vi "界面UI.vi"() -> ()   [LabVIEW 2016, in "德润DR803L超标留样.lvlib"]
uses:
  <vilib>/Utility/miscctls.llb/LVPointTypeDef.ctl
  <vilib>/Utility/config.llb/NI_LVConfig.lvlib
  <vilib>/ptbypt/NI_PtbyPt.lvlib
panel:
  in  "超标浓度配置":bool
  out "流程中":bool
  in  "停止流程":bool
  in  "启动流程":bool
  in  "时间等比采样":u16=10
  in  "单次采样量":u16=500
  in  "修改门禁密码":bool
  in  "远程复位":bool
  in  "排空当前瓶":bool
  in  "采样方式":enum16{"单采", "双重"}(ring)
  in  "远程留样":bool
  in  "选择留样瓶":bool
  in  "排空留样瓶":bool
  out "采样器状态":T1
  out "Registers":u16[](array[numeric])
  in  "打开串口":bool
  in  "释放串口":bool
  in  "留样模式":T2(ring)=enum."外控留样"
  in  "采样启动":bool
  in  "停止命令":bool
  in  "切换采样器状态":bool
  in  "时间校准":bool
  out "source":string
  out "通讯":bool
  # "只在停止时切换有效"
  # "只在待机时切换有效"
  # "默认：500ml（5-1000）ml （只在停止时写有效）"
  # "只在待机时启动有效"
  # "默认：10min（2-9999）min （只在停止时写有效）"
  # "只在待机时启动有效"
  # "只在待机时启动有效"
  # "德润DR803L超标留样"
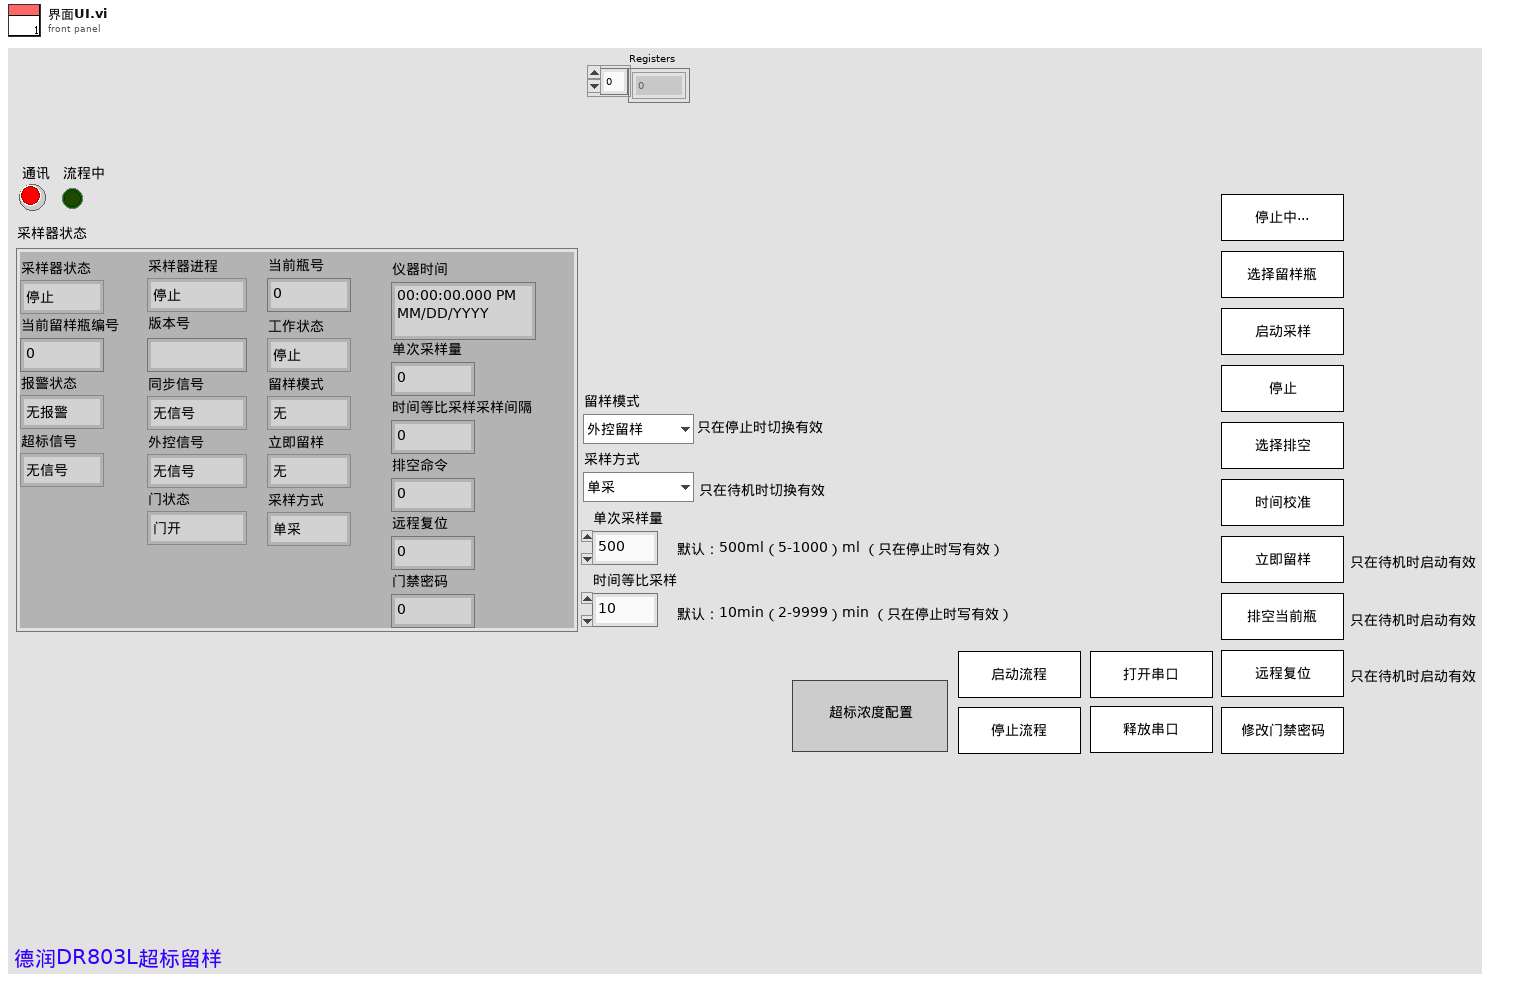
[diagram p1: front panel]
types:
  T1 = cluster{"采样器状态":enum16{"停止", "运行"}, "当前留样瓶编号":u16, "报警状态":enum16{"无报警", "缺水报警"}, "超标信号":enum16{"无信号", "超标信号"}, "采样器进程":enum16{"停止", "待机", "定位校正", "移除瓶盖", "采样瓶排空", "管路润洗", "管存", "进样", "瓶盖密封", "管路排空", "调整采样位置", "采样结束", "采样瓶润洗", "瓶润洗排空"}, "版本号":string, "同步信号":enum16{"无信号", "同步信号"}, "外控信号":enum16{"无信号", "外控信号"}, "门状态":enum16{"门开", "门关"}, "当前瓶号":u16, "工作状态":enum16{"停止", "采样中"}, "留样模式":enum16{"无", "定时留样", "时间等比例", "超标留样", "同步留样", "外控留样"}, "立即留样":enum16{"无", "远程留样"}, "采样方式":enum16{"单采", "双重"}, "仪器时间":timestamp, "单次采样量":u16, "时间等比采样采样间隔":u16, "排空命令":u16, "远程复位":u16, "门禁密码":u16}
  T2 = enum16{"无", "定时留样", "时间等比例", "超标留样", "同步留样", "外控留样"}
  T3 = cluster{"STEP":enum16{"open", "read", "write", "write single", "close"}, "starting address":u16, "value":u16}
  T4 = typedef "LVPointTypeDef.ctl" = cluster{"Horizontal":i16, "Vertical":i16}
  T5 = typedef "NI_LVConfig.lvlib/Config Data RefNum.ctl" = refnum<k1>
  T6 = enum16{"open", "read", "write", "write single", "close"}
  T7 = cluster{"氨氮超标浓度":dbl, "总磷超标浓度":dbl, "总氮超标浓度":dbl, "CODMn超标浓度":dbl, "CODCr超标浓度":dbl}
  T8 = typedef "LVDateTimeRec.ctl" = cluster{"秒数的小数部分":dbl, "秒":i32, "分":i32, "时":i32, "日":i32, "月":i32, "年":i32, "天数（周）":i32, "天数（年）":i32, "DST":i32}
  T9 = enum32{"Bad", "Idle", "Run top level", "Running"}
  T10 = cluster{"确定":bool, "氨氮超标浓度":dbl, "总磷超标浓度":dbl, "总氮超标浓度":dbl, "CODMn超标浓度":dbl, "CODCr超标浓度":dbl}
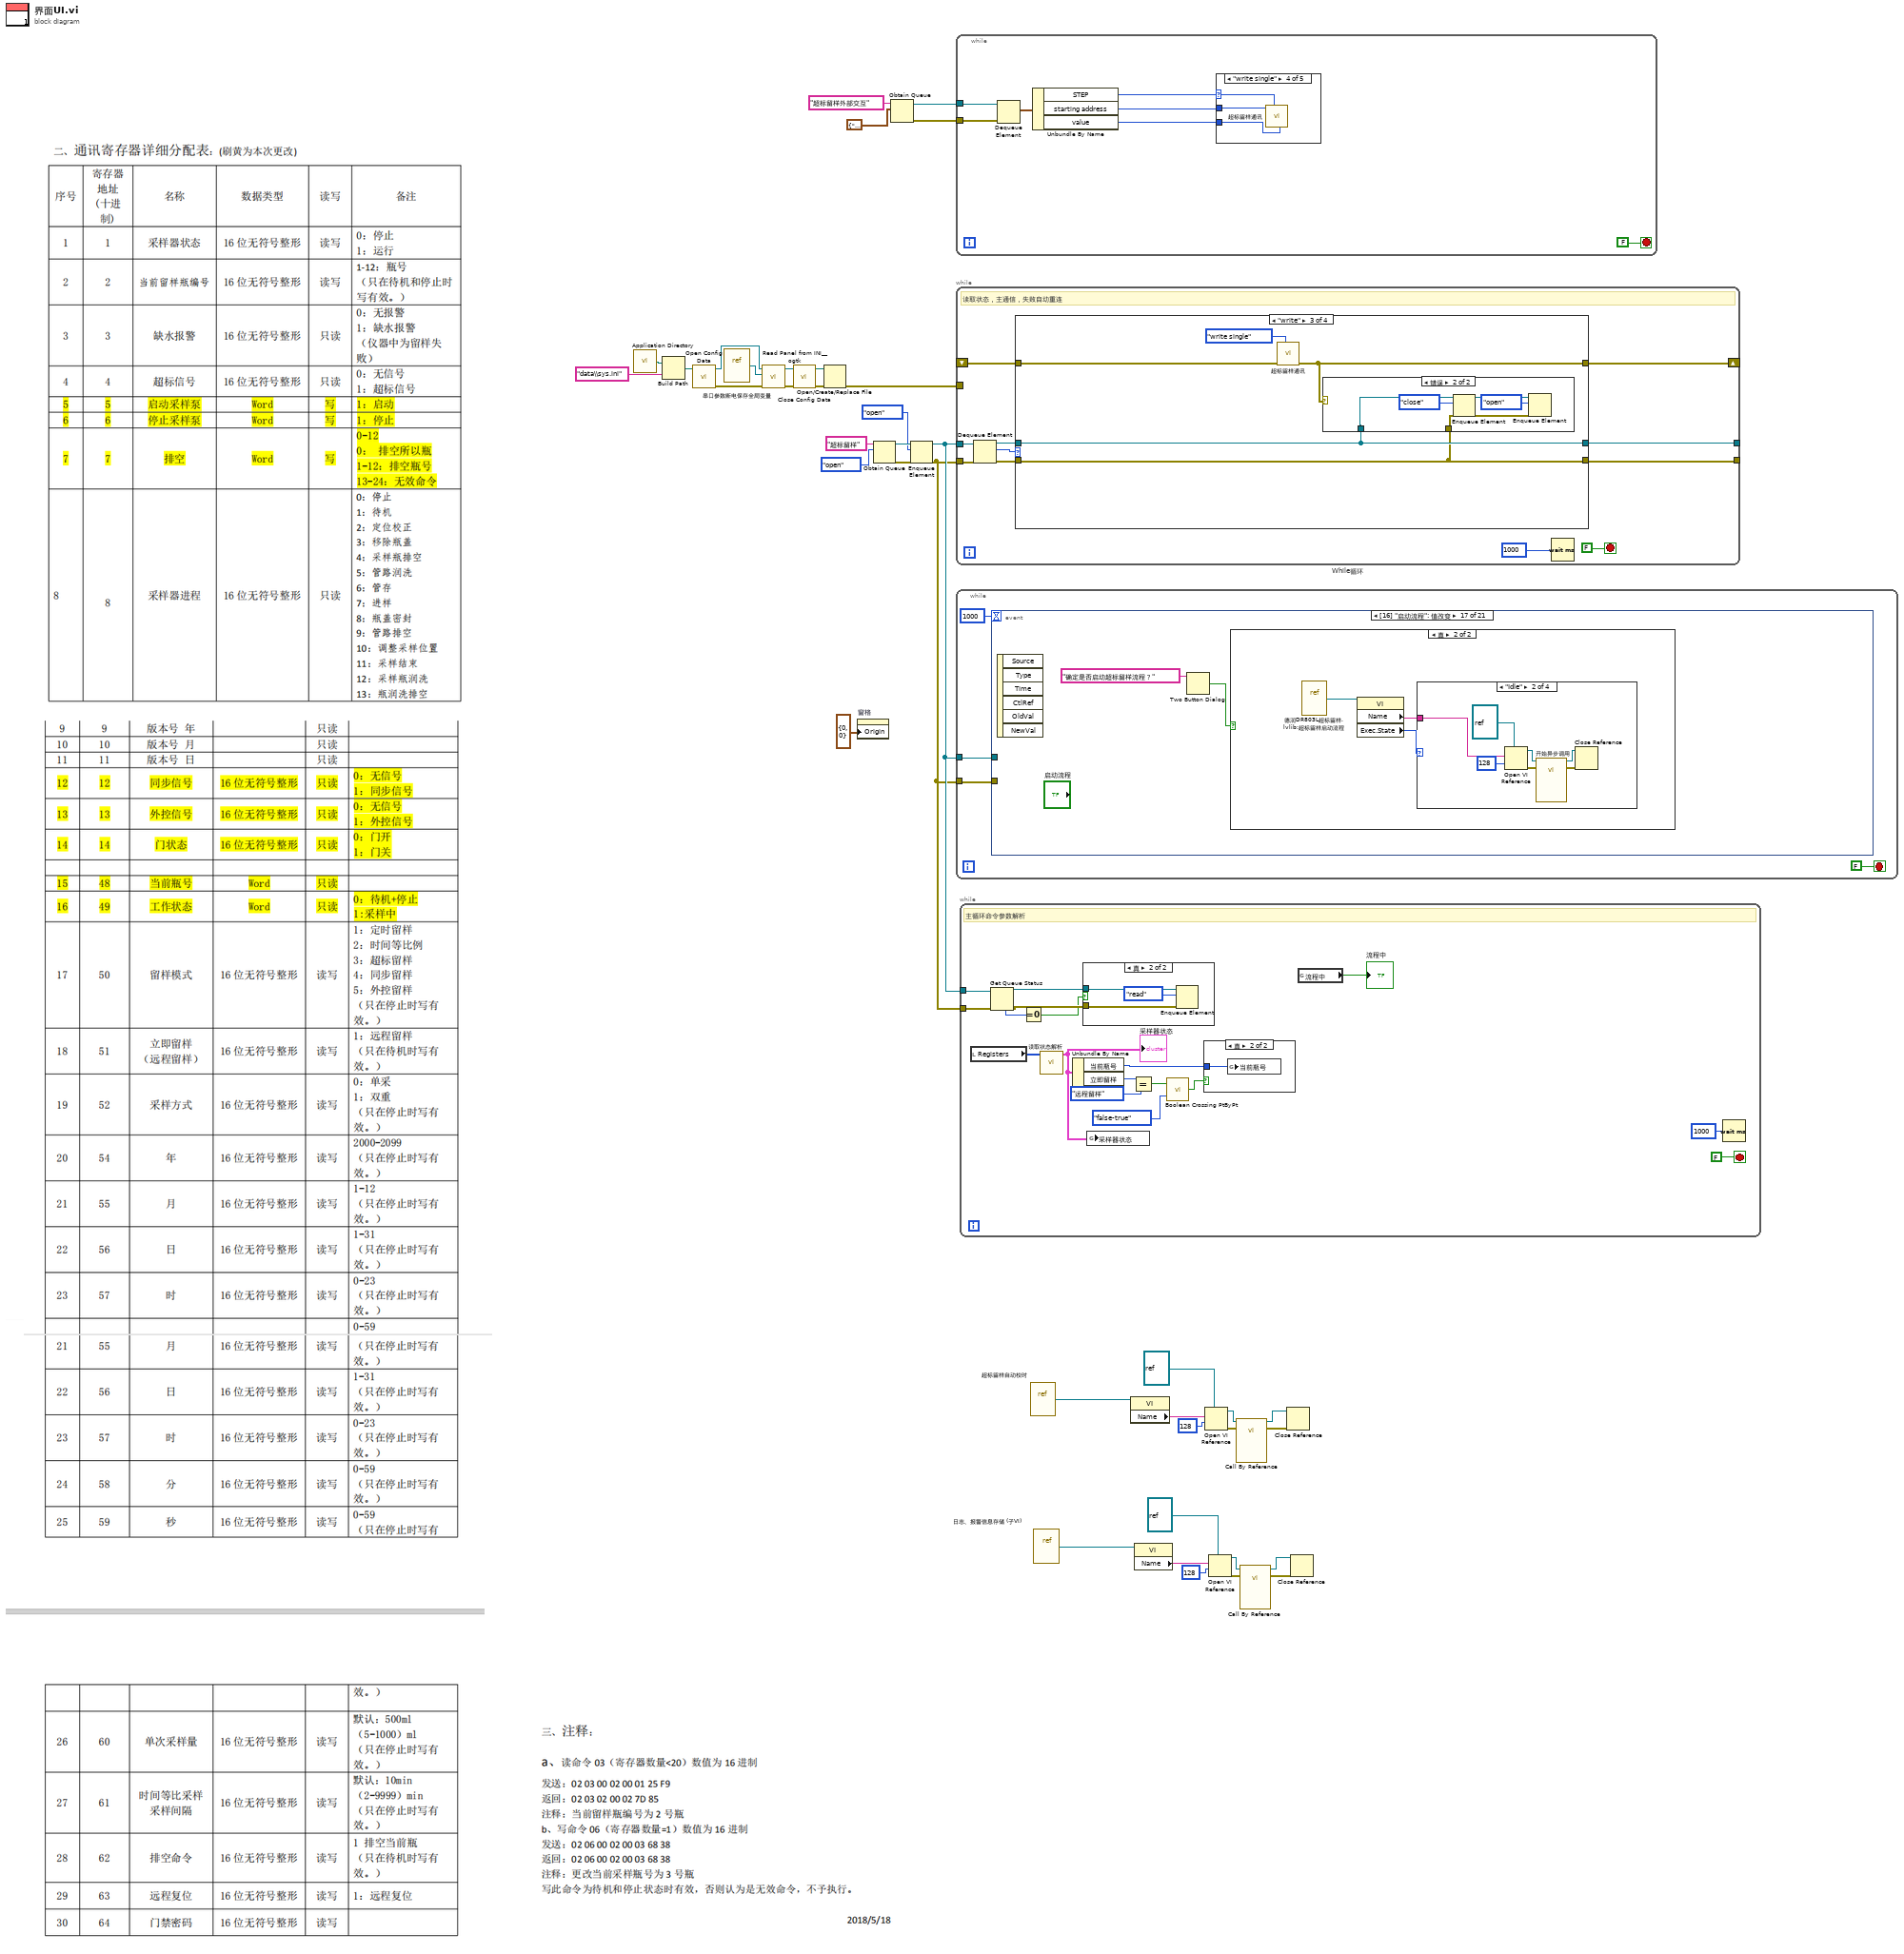
[diagram p0: block diagram]
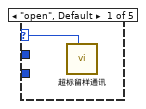
[diagram p2: hidden frame]
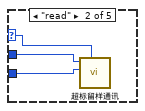
[diagram p3: hidden frame]
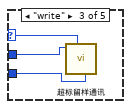
[diagram p4: hidden frame]
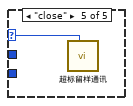
[diagram p5: hidden frame]
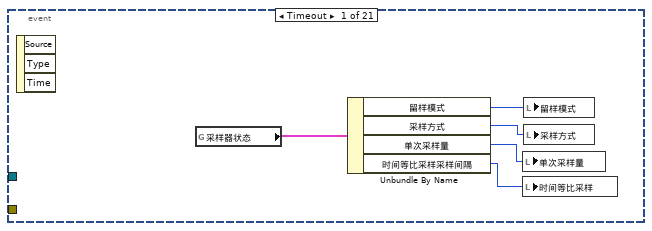
[diagram p6: hidden frame]
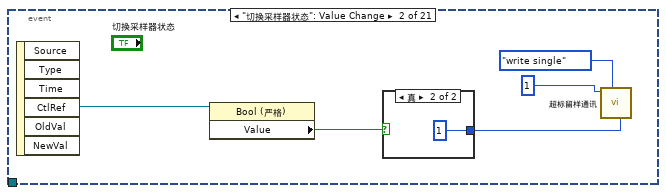
[diagram p7: hidden frame]
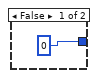
[diagram p8: hidden frame]
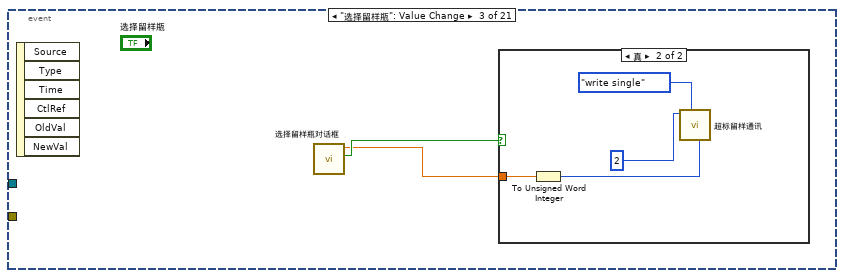
[diagram p9: hidden frame]
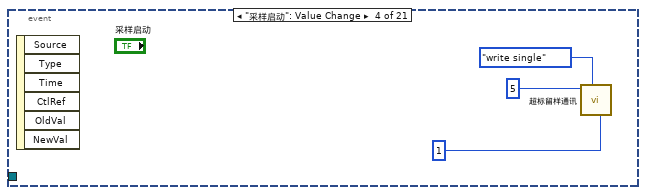
[diagram p11: hidden frame]
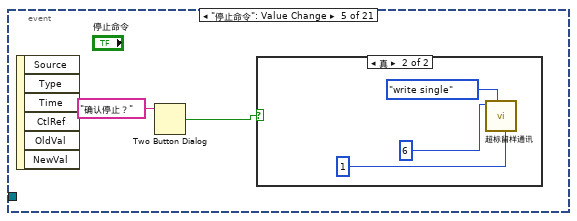
[diagram p12: hidden frame]
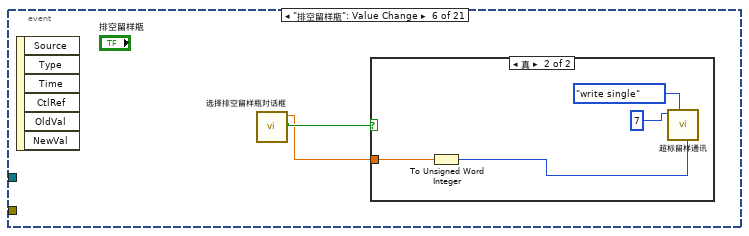
[diagram p14: hidden frame]
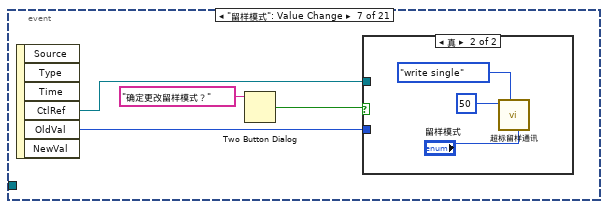
[diagram p16: hidden frame]
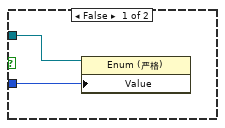
[diagram p17: hidden frame]
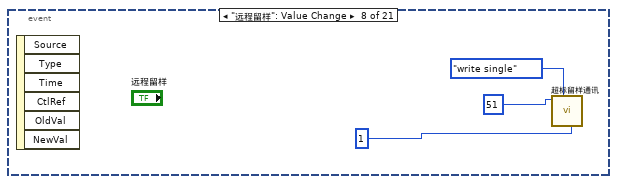
[diagram p18: hidden frame]
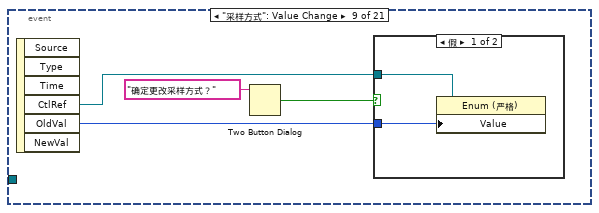
[diagram p19: hidden frame]
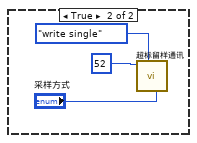
[diagram p20: hidden frame]
diagram:
  n1 = call <vilib>:"Application Directory.vi"() -> ("Application Directory"=w31:path)
  n2 = Build Path(base path=w31, name or relative path="data\\sys.ini" ("名称或相对路径")) -> (appended path=w29:path)
  n3 = call <vilib>:"Open Config Data.vi"("configuration file path"=w29) -> ("error out"=w25:errorcluster, "refnum"=w28:T5)  [unwired: 8 in, 1 out]
  n4 = vi-ref "串口参数断电保存全局变量.vi"() -> (w27:refnum<vi>)
  n5 = call <userlib>:"Read Panel from INI__ogtk.vi"("error in (no error)"=w25, "VI ref"=w27, "refnum"=w28) -> ("error out"=w24:errorcluster, "refnum out"=w26:T5)  [unwired: 7 in]
  n6 = call <vilib>:"Close Config Data.vi"("error in (no error)"=w24, "refnum"=w26) -> ("error out"=w23:errorcluster, "file path"=w22:path)  [unwired: 8 in]
  n7 = Open/Create/Replace File(file path (use dialog)=w22, error in=w23) -> (error out=w21:errorcluster)  [unwired: 4 in, 2 out]
  n8 = property on="窗格" class="Pane"("Origin"=T4 {"Horizontal"=0, "Vertical"=0} ("原点")) -> ()  [unwired: 2 in, 2 out]
  n9 = Obtain Queue(name (unnamed)="超标留样" ("名称（未命名）"), element data type=enum16{"open", "read", "write", "close"}."open") -> (queue out=w37:refnum<queue>, error out=w36:errorcluster)  [unwired: 3 in, 1 out]
  n10 = Obtain Queue(name (unnamed)="超标留样外部交互" ("名称（未命名）"), element data type=T3 {"STEP"=enum."write single", "starting address"=0, "value"=0}) -> (queue out=w18:refnum<queue>, error out=w17:errorcluster)  [unwired: 3 in, 1 out]
  n11 = Enqueue Element(queue=w37, element=enum16{"open", "read", "write", "close"}."open", error in (no error)=w36) -> (queue out=w34:refnum<queue>, error out=w33:errorcluster)  [unwired: 1 in, 1 out]
  n12 = while {
    tunnel: w34 -> [w42]
    tunnel: w33 -> [w41]
    stop <- FALSE stop-if-true
    n13 = event shown="[16] \"启动流程\": 值改变" {
      selector: _ -> [_ _ _ _ _ _ _ _ _ _ _ _ _ _ _ _ _ _ _ _ _]
      dyn-events: _ -> [_ _ _ _ _ _ _ _ _ _ _ _ _ _ _ _ _ _ _ _ _]
      timeout: 1000 -> [_ _ _ _ _ _ _ _ _ _ _ _ _ _ _ _ _ _ _ _ _]
      tunnel: w42 -> [_ _ _ _ _ _ _ _ _ _ _ _ _ _ _ _ _ _ w172 w178 _]
      tunnel: w41 -> [_ _ _ _ _ _ _ _ _ _ _ _ _ _ _ _ _ _ w171 w177 _]
      event Timeout {
        n14 = event-data() -> ()  [unwired: 1 in, 3 out]
        n15 = global read "超标留样全局.vi" "采样器状态"() -> (w44:T1)
        n16 = Unbundle By Name(w44) -> ("留样模式"=w48:T2, "采样方式"=w45:enum16{"单采", "双重"}, "单次采样量"=w46:u16, "时间等比采样采样间隔"=w47:u16)
        n17 = local write "单次采样量"(w46) -> ()
        n18 = local write "时间等比采样"(w47) -> ()
        n19 = local write "留样模式"(w48) -> ()
        n20 = local write "采样方式"(w45) -> ()
      }
      event "切换采样器状态": Value Change {
        n21 = event-data() -> ("CtlRef"=w53:refnum<vi>)  [unwired: 1 in, 5 out]
        n22 = property class="Bool (严格)"(reference=w53) -> ("Value"=w52:bool)  [unwired: 1 in, 2 out]
        n23 = case shown="真" w52 {
          tunnel: [u16 0 ("索引") u16 1 ("索引")] -> w49
          frame False {
          }
          frame True {
          }
        }
        n24 = call "超标留样通讯.vi"("value"=w49, "STEP"=T6."write single", "starting address"=1 ("索引")) -> ()  [unwired: 6 in, 3 out]
      }
      event "选择留样瓶": Value Change {
        n25 = event-data() -> ()  [unwired: 1 in, 6 out]
        n26 = call "选择留样瓶对话框.vi"() -> ("布尔"=w57:bool, "选择留样瓶"=w56:dbl)  [unwired: 10 in]
        n27 = case shown="真" w57 {
          tunnel: w56 -> [_ w58]
          frame False {
          }
          frame True {
            n28 = To Unsigned Word Integer(number=w58) -> (unsigned 16bit integer=w59:u16)
            n29 = call "超标留样通讯.vi"("value"=w59, "STEP"=T6."write single", "starting address"=2 ("索引")) -> ()  [unwired: 6 in, 3 out]
          }
        }
      }
      event "采样启动": Value Change {
        n30 = event-data() -> ()  [unwired: 1 in, 6 out]
        n31 = call "超标留样通讯.vi"("value"=u16 1 ("新元素/子数组"), "STEP"=T6."write single", "starting address"=5 ("索引")) -> ()  [unwired: 6 in, 3 out]
      }
      event "停止命令": Value Change {
        n32 = event-data() -> ()  [unwired: 1 in, 6 out]
        n33 = Two Button Dialog(message="确认停止？" ("消息")) -> (T button?=w65:bool)  [unwired: 2 in]
        n34 = case shown="真" w65 {
          frame False {
          }
          frame True {
            n35 = call "超标留样通讯.vi"("value"=u16 1 ("新元素/子数组"), "STEP"=T6."write single", "starting address"=6 ("索引")) -> ()  [unwired: 6 in, 3 out]
          }
        }
      }
      event "排空留样瓶": Value Change {
        n36 = event-data() -> ()  [unwired: 1 in, 6 out]
        n37 = call "选择排空留样瓶对话框.vi"() -> ("布尔"=w71:bool, "选择留样瓶"=w70:dbl)  [unwired: 10 in]
        n38 = case shown="真" w71 {
          tunnel: w70 -> [_ w75]
          frame False {
          }
          frame True {
            n39 = To Unsigned Word Integer(number=w75) -> (unsigned 16bit integer=w72:u16)
            n40 = call "超标留样通讯.vi"("value"=w72, "STEP"=T6."write single", "starting address"=7 ("索引")) -> ()  [unwired: 6 in, 3 out]
          }
        }
      }
      event "留样模式": Value Change {
        n41 = event-data() -> ("CtlRef"=w76:refnum<vi>, "OldVal"=w77:T2)  [unwired: 1 in, 4 out]
        n42 = Two Button Dialog(message="确定更改留样模式？" ("消息")) -> (T button?=w78:bool)  [unwired: 2 in]
        n43 = case shown="真" w78 {
          tunnel: w77 -> [w80 _]
          tunnel: w76 -> [w81 _]
          frame False {
            n44 = property class="Enum (严格)"(reference=w81, "Value"=w80) -> ()  [unwired: 1 in, 2 out]
          }
          frame True {
            n45 = call "超标留样通讯.vi"("value"="留样模式", "STEP"=T6."write single", "starting address"=50 ("索引")) -> ()  [unwired: 6 in, 3 out]
          }
        }
      }
      event "远程留样": Value Change {
        n46 = event-data() -> ()  [unwired: 1 in, 6 out]
        n47 = call "超标留样通讯.vi"("value"=u16 1 ("新元素/子数组"), "STEP"=T6."write single", "starting address"=51 ("索引")) -> ()  [unwired: 6 in, 3 out]
      }
      event "采样方式": Value Change {
        n48 = event-data() -> ("CtlRef"=w89:refnum<vi>, "OldVal"=w88:enum16{"单采", "双重"})  [unwired: 1 in, 4 out]
        n49 = Two Button Dialog(message="确定更改采样方式？" ("消息")) -> (T button?=w90:bool)  [unwired: 2 in]
        n50 = case shown="假" w90 {
          tunnel: w89 -> [w93 _]
          tunnel: w88 -> [w92 _]
          frame False {
            n51 = property class="Enum (严格)"(reference=w93, "Value"=w92) -> ()  [unwired: 1 in, 2 out]
          }
          frame True {
            n52 = call "超标留样通讯.vi"("value"="采样方式", "STEP"=T6."write single", "starting address"=52 ("索引")) -> ()  [unwired: 6 in, 3 out]
          }
        }
      }
      event "时间校准": Value Change {
        n53 = event-data() -> ()  [unwired: 1 in, 6 out]
        n54 = Get Date/Time In Seconds() -> (seconds since 1Jan1904=w109:timestamp)
        n55 = Seconds To Date/Time(time stamp (now)=w109) -> (date time rec=w108:T8)  [unwired: 1 in]
        n56 = Unbundle By Name(w108) -> ("年"=w105:i32, "月"=w104:i32, "日"=w103:i32, "时"=w102:i32, "分"=w101:i32, "秒"=w100:i32)
        n57 = Build Array(w105, w104, w103, w102, w101, w100) -> (w99:i32[])
        n58 = Insert Into Array(array=u16[] [] ("values"), new element=w99) -> (w106:u16[])  [unwired: 1 in]
        n59 = call "超标留样通讯.vi"("STEP"=T6."write", "values"=w106, "starting address"=54 ("索引")) -> ()  [unwired: 6 in, 3 out]
      }
      event "单次采样量", "时间等比采样": Mouse Down {
        n60 = event-data() -> ("CtlRef"=w113:refnum<vi>)  [unwired: 1 in, 7 out]
        n61 = property class="DigNum (严格)"(reference=w113) -> (reference out=w112:refnum<vi>, "Value"=w111:u16)  [unwired: 1 in, 1 out]
        n62 = call "数字键盘.vi"("OldNumber"=w111) -> ("NewNumber"=w110:sgl)
        n63 = property class="DigNum (严格)"(reference=w112, "Val(Sgnl)"=w110) -> ()  [unwired: 1 in, 2 out]
      }
      event "单次采样量": Value Change {
        n64 = event-data() -> ()  [unwired: 1 in, 6 out]
        n65 = call "超标留样通讯.vi"("value"="单次采样量", "STEP"=T6."write single", "starting address"=60 ("索引")) -> ()  [unwired: 6 in, 3 out]
      }
      event "时间等比采样": Value Change {
        n66 = event-data() -> ()  [unwired: 1 in, 6 out]
        n67 = call "超标留样通讯.vi"("value"="时间等比采样", "STEP"=T6."write single", "starting address"=61 ("索引")) -> ()  [unwired: 6 in, 3 out]
      }
      event "排空当前瓶": Value Change {
        n68 = event-data() -> ()  [unwired: 1 in, 6 out]
        n69 = Two Button Dialog(message="是否排空当前瓶？" ("消息")) -> (T button?=w120:bool)  [unwired: 2 in]
        n70 = case shown="真" w120 {
          frame False {
          }
          frame True {
            n71 = call "超标留样通讯.vi"("value"=u16 1 ("新元素/子数组"), "STEP"=T6."write single", "starting address"=63 ("索引")) -> ()  [unwired: 6 in, 3 out]
          }
        }
      }
      event "远程复位": Value Change {
        n72 = event-data() -> ()  [unwired: 1 in, 6 out]
        n73 = Two Button Dialog(message="确认复位？" ("消息")) -> (T button?=w125:bool)  [unwired: 2 in]
        n74 = case shown="真" w125 {
          frame False {
          }
          frame True {
            n75 = call "超标留样通讯.vi"("value"=u16 1 ("新元素/子数组"), "STEP"=T6."write single", "starting address"=64 ("索引")) -> ()  [unwired: 6 in, 3 out]
          }
        }
      }
      event "修改门禁密码": Value Change {
        n76 = event-data() -> ()  [unwired: 1 in, 6 out]
        n77 = Two Button Dialog(message="确定修改门禁密码？" ("消息")) -> (T button?=w130:bool)  [unwired: 2 in]
        n78 = case shown="真" w130 {
          frame False {
          }
          frame True {
            n79 = local read "采样器状态"() -> (w133:T1)
            n80 = Unbundle By Name(w133) -> ("门禁密码"=w132:u16)
            n81 = call "数字键盘.vi"("OldNumber"=w132) -> ("NewNumber"=w136:sgl)
            n82 = Less?(x=w136, y=sgl 65535.0) -> (x < y?=w134:bool)
            n83 = case shown="真" w134 {
              tunnel: w136 -> [_ w140]
              frame False {
              }
              frame True {
                n84 = To Unsigned Word Integer(number=w140) -> (unsigned 16bit integer=w137:u16)
                n85 = call "超标留样通讯.vi"("value"=w137, "STEP"=T6."write single", "starting address"=65 ("索引")) -> ()  [unwired: 6 in, 3 out]
              }
            }
          }
        }
      }
      event "启动流程": Value Change {
        n86 = event-data() -> ()  [unwired: 1 in, 6 out]
        n87 = Two Button Dialog(message="确定是否启动超标留样流程？" ("消息")) -> (T button?=w141:bool)  [unwired: 2 in]
        n88 = case shown="真" w141 {
          frame False {
          }
          frame True {
            n89 = vi-ref "德润DR803L超标留样.lvlib:超标留样启动流程.vi"() -> (w143:refnum<vi>)
            n90 = property class="VI"(reference=w143) -> ("Name"=w144:string, "Exec.State"=w145:T9)  [unwired: 1 in, 2 out]
            n91 = case shown="\"Idle\"" w145 {
              tunnel: w144 -> [_ w148 _ _]
              frame "Bad", Default {
              }
              frame "Idle" {
                n92 = Open VI Reference(type specifier VI Refnum (for type only)=refnum<vi> refnum ("类型说明符VI引用句柄（仅用于类型）"), vi path=w148, options=128 ("选项")) -> (vi reference=w152:refnum<vi>, error out=w147:errorcluster)  [unwired: 3 in]
                n93 = call-by-ref "开始异步调用"(reference=w152, error in=w147) -> (reference out=w151:refnum<vi>, error out=w146:errorcluster)  [unwired: 12 in]
                n94 = Close Reference(reference=w151, error in (no error)=w146) -> ()  [unwired: 1 out]
              }
              frame "Run top level" {
              }
              frame "Running" {
                n95 = One Button Dialog(message="流程已启动，无需重复启动！" ("消息")) -> ()  [unwired: 1 in, 1 out]
              }
            }
          }
        }
      }
      event "停止流程": Value Change {
        n96 = event-data() -> ()  [unwired: 1 in, 6 out]
        n97 = Two Button Dialog(message="确定是否停止超标留样流程并排空当前瓶？" ("消息")) -> (T button?=w154:bool)  [unwired: 2 in]
        n98 = case shown="真" w154 {
          frame False {
          }
          frame True {
            n99 = Obtain Notifier(name (unnamed)="超标留样流程" ("名称（未命名）"), notification data type=FALSE ("采样完成")) -> (notifier out=w167:refnum<notifier>, error out=w166:errorcluster)  [unwired: 2 in, 1 out]
            n100 = Send Notification(notification=TRUE ("通知"), notifier=w167, error in (no error)=w166) -> (notifier out=w164:refnum<notifier>, error out=w163:errorcluster)
            n101 = call "超标留样通讯.vi"("value"=u16 1 ("新元素/子数组"), "STEP"=T6."write single", "starting address"=6 ("索引")) -> ("error out"=w156:errorcluster)  [unwired: 6 in, 2 out]
            n102 = Release Notifier(notifier=w164, error in (no error)=w163) -> ()  [unwired: 1 in, 3 out]
            n103 = call "超标留样通讯.vi"("value"=u16 1 ("新元素/子数组"), "STEP"=T6."write single", "Error in"=w156, "starting address"=63 ("索引")) -> ()  [unwired: 5 in, 3 out]
          }
        }
      }
      event "释放串口": Value Change {
        n104 = event-data() -> ()  [unwired: 1 in, 6 out]
        n105 = Two Button Dialog(message="确认是否释放串口，释放串口将导致通信失败！" ("消息")) -> (T button?=w170:bool)  [unwired: 2 in]
        n106 = case shown="真" w170 {
          tunnel: w172 -> [_ w175]
          tunnel: w171 -> [_ w174]
          frame False {
          }
          frame True {
            n107 = Enqueue Element(queue=w175, element=enum16{"open", "read", "write", "close"}."close" ("元素"), error in (no error)=w174) -> ()  [unwired: 1 in, 3 out]
          }
        }
      }
      event "打开串口": Value Change {
        n108 = event-data() -> ()  [unwired: 1 in, 6 out]
        n109 = global read "串口参数断电保存全局变量.vi" "VISA resource name"() -> (w186:refnum<visa-resource-name>)
        n110 = global read "串口参数断电保存全局变量.vi" "MB通信方式选择"() -> (w187:enum16{"串口", "TCP"})
        n111 = global read "串口参数断电保存全局变量.vi" "PORT"() -> (w184:string)
        n112 = global read "串口参数断电保存全局变量.vi" "IP"() -> (w185:string)
        n113 = call "串口配置.vi"("PORT"=w184, "IP"=w185, "MB通信方式选择"=w187, "请选择串口:"=w186) -> ("PORT 2"=w180:string, "IP 2"=w181:string, "确认 2"=w183:bool, "VISA资源名称 2"=w182:refnum<visa-resource-name>, "MB通信方式选择 2"=w179:enum16{"串口", "TCP"})  [unwired: 3 in]
        n114 = case shown="真" w183 {
          tunnel: w182 -> [_ w195]
          tunnel: w181 -> [_ w194]
          tunnel: w180 -> [_ w193]
          tunnel: w179 -> [_ w192]
          tunnel: w178 -> [_ w191]
          tunnel: w177 -> [_ w189]
          frame False {
          }
          frame True {
            n115 = flat-sequence {
              tunnel: w195 -> [w201]
              tunnel: w194 -> [w200]
              tunnel: w193 -> [w199]
              tunnel: w192 -> [w198]
              tunnel: w191 -> [w197]
              tunnel: [w197] -> w190
              tunnel: w189 -> [w196]
              tunnel: [w196] -> w188
              tunnel: w190 -> [w203]
              tunnel: w188 -> [w202]
              frame #0 {
                n116 = global write "串口参数断电保存全局变量.vi" "VISA resource name"(w201) -> ()
                n117 = global write "串口参数断电保存全局变量.vi" "MB通信方式选择"(w198) -> ()
                n118 = global write "串口参数断电保存全局变量.vi" "PORT"(w199) -> ()
                n119 = global write "串口参数断电保存全局变量.vi" "IP"(w200) -> ()
              }
              frame #1 {
                n120 = call <vilib>:"Application Directory.vi"() -> ("Application Directory"=w206:path)
                n121 = Build Path(base path=w206, name or relative path="data\\sys.ini" ("名称或相对路径")) -> (appended path=w207:path)
                n122 = Enqueue Element(queue=w203, element=enum16{"open", "read", "write", "close"}."open" ("元素"), error in (no error)=w202) -> ()  [unwired: 1 in, 3 out]
                n123 = call <vilib>:"Open Config Data.vi"("configuration file path"=w207) -> ("error out"=w211:errorcluster, "refnum"=w208:T5)  [unwired: 8 in, 1 out]
                n124 = vi-ref "串口参数断电保存全局变量.vi"() -> (w209:refnum<vi>)
                n125 = call <userlib>:"Write Panel to INI__ogtk.vi"("error in (no error)"=w211, "VI ref"=w209, "refnum"=w208) -> ("error out"=w212:errorcluster, "refnum out"=w210:T5)  [unwired: 7 in]
                n126 = call <vilib>:"Close Config Data.vi"("error in (no error)"=w212, "refnum"=w210) -> ("error out"=w217:errorcluster, "file path"=w218:path)  [unwired: 8 in]
                n127 = Open/Create/Replace File(file path (use dialog)=w218, error in=w217) -> (refnum out=w214:refnum<file>, error out=w213:errorcluster)  [unwired: 4 in, 1 out]
                n128 = Flush File(refnum=w214, error in=w213) -> (refnum out=w215:refnum<file>, error out=w216:errorcluster)
                n129 = Close File(refnum=w215, error in=w216) -> ()  [unwired: 2 out]
              }
            }
          }
        }
      }
      event "超标浓度配置": Value Change {
        n130 = event-data() -> ()  [unwired: 1 in, 6 out]
        n131 = global read "串口参数断电保存全局变量.vi" "CODMn超标浓度"() -> (w230:dbl)
        n132 = global read "串口参数断电保存全局变量.vi" "CODCr超标浓度"() -> (w229:dbl)
        n133 = global read "串口参数断电保存全局变量.vi" "总磷超标浓度"() -> (w227:dbl)
        n134 = global read "串口参数断电保存全局变量.vi" "总氮超标浓度"() -> (w231:dbl)
        n135 = global read "串口参数断电保存全局变量.vi" "氨氮超标浓度"() -> (w228:dbl)
        n136 = Bundle By Name(cluster=T7 {"氨氮超标浓度"=0.0, "总磷超标浓度"=0.0, "总氮超标浓度"=0.0, "CODMn超标浓度"=0.0, "CODCr超标浓度"=0.0} ("输入"), "氨氮超标浓度"=w228, "总磷超标浓度"=w227, "总氮超标浓度"=w231, "CODMn超标浓度"=w230, "CODCr超标浓度"=w229) -> (w226:T7)
        n137 = call "超标浓度设置.vi"("输入"=w226) -> ("输出"=w225:T10)  [unwired: 10 in]
        n138 = Unbundle By Name(w225) -> ("确定"=w224:bool, "氨氮超标浓度"=w223:dbl, "总磷超标浓度"=w222:dbl, "总氮超标浓度"=w221:dbl, "CODMn超标浓度"=w220:dbl, "CODCr超标浓度"=w219:dbl)
        n139 = case shown="真" w224 {
          tunnel: w223 -> [_ w237]
          tunnel: w222 -> [_ w236]
          tunnel: w221 -> [_ w235]
          tunnel: w220 -> [_ w234]
          tunnel: w219 -> [_ w233]
          frame False {
          }
          frame True {
            n140 = flat-sequence {
              tunnel: w237 -> [w242]
              tunnel: w236 -> [w241]
              tunnel: w235 -> [w240]
              tunnel: w234 -> [w239]
              tunnel: w233 -> [w238]
              frame #0 {
                n141 = global write "串口参数断电保存全局变量.vi" "CODMn超标浓度"(w239) -> ()
                n142 = global write "串口参数断电保存全局变量.vi" "CODCr超标浓度"(w238) -> ()
                n143 = global write "串口参数断电保存全局变量.vi" "总磷超标浓度"(w241) -> ()
                n144 = global write "串口参数断电保存全局变量.vi" "总氮超标浓度"(w240) -> ()
                n145 = global write "串口参数断电保存全局变量.vi" "氨氮超标浓度"(w242) -> ()
              }
              frame #1 {
                n146 = call <vilib>:"Application Directory.vi"() -> ("Application Directory"=w244:path)
                n147 = Build Path(base path=w244, name or relative path="data\\sys.ini" ("名称或相对路径")) -> (appended path=w245:path)
                n148 = call <vilib>:"Open Config Data.vi"("configuration file path"=w245) -> ("error out"=w249:errorcluster, "refnum"=w246:T5)  [unwired: 8 in, 1 out]
                n149 = vi-ref "串口参数断电保存全局变量.vi"() -> (w247:refnum<vi>)
                n150 = call <userlib>:"Write Panel to INI__ogtk.vi"("error in (no error)"=w249, "VI ref"=w247, "refnum"=w246) -> ("error out"=w250:errorcluster, "refnum out"=w248:T5)  [unwired: 7 in]
                n151 = call <vilib>:"Close Config Data.vi"("error in (no error)"=w250, "refnum"=w248) -> ("error out"=w255:errorcluster, "file path"=w256:path)  [unwired: 8 in]
                n152 = Open/Create/Replace File(file path (use dialog)=w256, error in=w255) -> (refnum out=w252:refnum<file>, error out=w251:errorcluster)  [unwired: 4 in, 1 out]
                n153 = Flush File(refnum=w252, error in=w251) -> (refnum out=w253:refnum<file>, error out=w254:errorcluster)
                n154 = Close File(refnum=w253, error in=w254) -> ()  [unwired: 2 out]
              }
            }
          }
        }
      }
    }
  }
  n155 = while {
    tunnel: w18 -> [w262]
    tunnel: w17 -> [w261]
    stop <- FALSE stop-if-true
    n156 = Dequeue Element(queue=w262, error in (no error)=w261) -> (element=w260:T3)  [unwired: 1 in, 3 out]
    n157 = Unbundle By Name(w260) -> ("STEP"=w259:T6, "starting address"=w258:u16, "value"=w257:u16)
    n158 = case shown="\"write single\"" w259 {
      selector: w259 -> [w264 w267 w270 w273 w274]
      tunnel: w258 -> [_ w266 w269 w272 _]
      tunnel: w257 -> [_ w265 w268 w271 _]
      frame "open", Default {
        n159 = call "超标留样通讯.vi"("STEP"=w264) -> ()  [unwired: 8 in, 3 out]
      }
      frame "read" {
        n160 = call "超标留样通讯.vi"("STEP"=w267, "quantity"=w265, "starting address"=w266) -> ()  [unwired: 6 in, 3 out]
      }
      frame "write" {
        n161 = call "超标留样通讯.vi"("value"=w268, "STEP"=w270, "starting address"=w269) -> ()  [unwired: 6 in, 3 out]
      }
      frame "write single" {
        n162 = call "超标留样通讯.vi"("value"=w271, "STEP"=w273, "starting address"=w272) -> ()  [unwired: 6 in, 3 out]
      }
      frame "close" {
        n163 = call "超标留样通讯.vi"("STEP"=w274) -> ()  [unwired: 8 in, 3 out]
      }
    }
  }
  n164 = while "While循环" {
    tunnel: w34 -> [w276]
    tunnel: w33 -> [w275]
    tunnel: [w280] -> _
    tunnel: [w279] -> _
    shift-right: [w277] -> _
    shift-left: _ -> [w278]
    tunnel: w21 -> [_]
    stop <- FALSE stop-if-true
    # "读取状态，主通信，失败自动重连"
    n165 = Dequeue Element(queue=w276, error in (no error)=w275) -> (queue out=w282:refnum<queue>, element=w283:enum16{"open", "read", "write", "close"}, error out=w281:errorcluster)  [unwired: 1 in, 1 out]
    n166 = case shown="\"write\"" w283 {
      tunnel: [w291 w293 w312 w321] -> w277
      tunnel: w282 -> [w290 w297 w311 w324]
      tunnel: w281 -> [w289 w296 w310 w323]
      tunnel: [w290 w297 w311 w324] -> w280
      tunnel: [w289 w296 w310 w323] -> w279
      tunnel: w278 -> [w288 w302 w314 w325]
      frame "open", Default {
        n167 = call "超标留样通讯.vi"("STEP"=T6."open", "Error in"=w288) -> ("error out"=w291:errorcluster, "MB session in"=w287:refnum<class "MB_Master.lvclass">)  [unwired: 7 in, 1 out]
        n168 = global write "串口参数断电保存全局变量.vi" "MB session in"(w287) -> ()
      }
      frame "read" {
        n169 = call "超标留样通讯.vi"("STEP"=T6."read", "Error in"=w302, "quantity"=u16 70, "starting address"=u16 0) -> ("error out"=w293:errorcluster, "Registers"=w299:u16[])  [unwired: 5 in, 1 out]
        n170 = Unbundle By Name(w293) -> ("status"=w295:bool, "source"=→"source":string)
        n171 = Not(x=w295) -> (.not. x?=w292:bool)
        "通讯" <- w292
        n172 = global write "超标留样全局.vi" "通讯"(w292) -> ()
        n173 = case shown="无错误" w293 {
          tunnel: w299 -> [w303 _]
          tunnel: w297 -> [_ w308]
          tunnel: w296 -> [_ w307]
          frame No Error {
            "Registers" <- w303
          }
          frame Error {
            n174 = Enqueue Element(queue=w308, element=enum16{"open", "read", "write", "close"}."close" ("元素"), error in (no error)=w307) -> (queue out=w306:refnum<queue>, error out=w305:errorcluster)  [unwired: 1 in, 1 out]
            n175 = Enqueue Element(queue=w306, element=enum16{"open", "read", "write", "close"}."open" ("元素"), error in (no error)=w305) -> ()  [unwired: 1 in, 3 out]
          }
        }
      }
      frame "write" {
        n176 = call "超标留样通讯.vi"("STEP"=T6."write single", "Error in"=w314) -> ("error out"=w312:errorcluster)  [unwired: 7 in, 2 out]
        n177 = case shown="错误" w312 {
          tunnel: w311 -> [_ w316]
          tunnel: w310 -> [_ w315]
          frame No Error {
          }
          frame Error {
            n178 = Enqueue Element(queue=w316, element=enum16{"open", "read", "write", "close"}."close" ("元素"), error in (no error)=w315) -> (queue out=w319:refnum<queue>, error out=w318:errorcluster)  [unwired: 1 in, 1 out]
            n179 = Enqueue Element(queue=w319, element=enum16{"open", "read", "write", "close"}."open" ("元素"), error in (no error)=w318) -> ()  [unwired: 1 in, 3 out]
          }
        }
      }
      frame "close" {
        n180 = call "超标留样通讯.vi"("STEP"=T6."close", "Error in"=w325) -> ("error out"=w321:errorcluster)  [unwired: 7 in, 2 out]
      }
    }
    n181 = Wait (ms)(milliseconds to wait=u32 1000 ("等待时间（毫秒）")) -> ()  [unwired: 1 out]
  }
  n182 = while {
    tunnel: w34 -> [w340]
    tunnel: w33 -> [w339]
    stop <- FALSE stop-if-true
    # "主循环命令参数解析"
    n183 = local read "Registers"() -> (w334:u16[])
    n184 = Get Queue Status(queue=w340, error in (no error)=w339) -> (queue out=w337:refnum<queue>, error out=w336:errorcluster, # elements in queue=w338:i32)  [unwired: 1 in, 5 out]
    n185 = Equal To 0?(x=w338) -> (x = 0?=w335:bool)
    n186 = call "读取状态解析.vi"("Registers"=w334) -> ("采样器状态"=w327:T1)  [unwired: 9 in, 1 out]
    "采样器状态" <- w327
    n187 = Unbundle By Name(w327) -> ("当前瓶号"=w329:u16, "立即留样"=w333:enum16{"无", "远程留样"})
    n188 = case shown="真" w335 {
      tunnel: w337 -> [_ w345]
      tunnel: w336 -> [_ w344]
      frame False {
      }
      frame True {
        n189 = Enqueue Element(queue=w345, element=enum16{"open", "read", "write", "close"}."read" ("元素"), error in (no error)=w344) -> ()  [unwired: 1 in, 3 out]
      }
    }
    n190 = global write "超标留样全局.vi" "采样器状态"(w327) -> ()
    n191 = Equal?(x=w333, y=enum16{"无", "远程留样"}."远程留样") -> (x = y?=w332:bool)
    n192 = call <vilib>:"Boolean Crossing PtByPt.vi"("direction"=enum16{"either", "false-true", "true-false"}."false-true", "input"=w332) -> ("crossing"=w330:bool)  [unwired: 1 in]
    n193 = case shown="真" w330 {
      tunnel: w329 -> [_ w343]
      frame False {
      }
      frame True {
        n194 = global write "超标留样全局.vi" "当前瓶号"(w343) -> ()
      }
    }
    n195 = global read "串口参数断电保存全局变量.vi" "流程中"() -> (→"流程中":bool)
    n196 = Wait (ms)(milliseconds to wait=u32 1000 ("等待时间（毫秒）")) -> ()  [unwired: 1 out]
  }
  n197 = vi-ref "超标留样自动校时.vi"() -> (w8:refnum<vi>)
  n198 = vi-ref "日志、报警信息存储 (子VI).vi"() -> (w9:refnum<vi>)
  n199 = property class="VI"(reference=w8) -> ("Name"=w7:string)  [unwired: 1 in, 2 out]
  n200 = property class="VI"(reference=w9) -> ("Name"=w10:string)  [unwired: 1 in, 2 out]
  n201 = Open VI Reference(type specifier VI Refnum (for type only)=refnum<vi> refnum, vi path=w7, options=128 ("选项")) -> (vi reference=w5:refnum<vi>, error out=w3:errorcluster)  [unwired: 3 in]
  n202 = Open VI Reference(type specifier VI Refnum (for type only)=refnum<vi> refnum, vi path=w10, options=128 ("选项")) -> (vi reference=w12:refnum<vi>, error out=w14:errorcluster)  [unwired: 3 in]
  n203 = call-by-ref "?"(reference=w5, error in=w3) -> (reference out=w1:refnum<vi>, error out=w2:errorcluster)  [unwired: 12 in]
  n204 = call-by-ref "?"(reference=w12, error in=w14) -> (reference out=w16:refnum<vi>, error out=w15:errorcluster)  [unwired: 12 in]
  n205 = Close Reference(reference=w1, error in (no error)=w2) -> ()  [unwired: 1 out]
  n206 = Close Reference(reference=w16, error in (no error)=w15) -> ()  [unwired: 1 out]
